vi "Create Enumeration.vi"(7 "App":refnum<vi>, 8 "error in (no error)":errorcluster, 10 "Enumeration":T1, 11 "LV-Protoc in":refnum<class "LV-Protoc.lvclass">) -> (0 "error out":errorcluster, 3 "LV-Protoc out":refnum<class "LV-Protoc.lvclass">)   [LabVIEW 2020, in "LV-Protoc.lvlib" / "LV-Protoc.lvclass"]
uses:
  LV-Protoc.lvclass
  LV-Proto/Enumeration.ctl
  LV-Proto/Enum Value.ctl
  LV-Protoc.lvlib
  LV-Proto/LV-Proto.lvlib
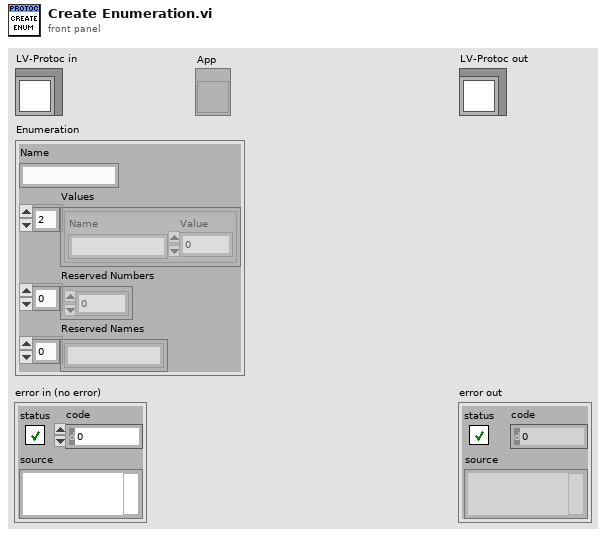
[diagram p1: front panel]
types:
  T1 = typedef "LV-Proto.lvlib/Enumeration.ctl" = cluster{"Name":string, "Values":T2[], "Reserved Numbers":u32[], "Reserved Names":string[]}
  T2 = typedef "LV-Proto.lvlib/Enum Value.ctl" = cluster{"Name":string, "Value":i32}
  T3 = typedef "LV-Protoc.lvlib/Enumeration Paths.ctl" = cluster{"Name":string, "Library":path, "Typedef":path, "Encode":path, "Encode packed":path, "Decode":path, "Decode packed":path, "Enum Value":path, "Enum from Value":path}
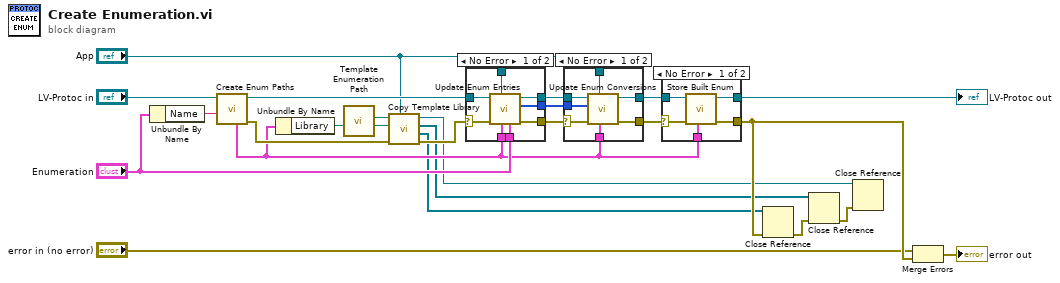
[diagram p0: block diagram]
diagram:
  n1 = Unbundle By Name("Enumeration") -> ("Name"=w14:string)
  n2 = call "Create Enum Paths.vi"("Enumeration Name"=w14, "LV-Protoc in"="LV-Protoc in") -> ("error out"=w13:errorcluster, "LV-Protoc out"=w15:refnum<class "LV-Protoc.lvclass">, "Enumeration Paths"=w8:T3)  [unwired: 7 in]
  n3 = Unbundle By Name(w8) -> ("Library"=w12:path)
  n4 = call "Template Enumeration Path.vi"() -> ("Template Enumeration Path"=w23:path)  [unwired: 11 in]
  n5 = call "Copy Template Library.vi"("App"="App", "error in (no error)"=w13, "Destination lvlib Path"=w12, "Source lvlib Path"=w23) -> ("error out"=w22:errorcluster, "Nested Libraries"=w5:refnum<vi>[], "VIs"=w3:refnum<vi>[], "Library"=w1:refnum<vi>)  [unwired: 4 in]
  n6 = case shown="No Error" w22 {
    selector: w22 -> [w30 w33]
    tunnel: w15 -> [w32 w34]
    tunnel: [w31 w34] -> w18
    tunnel: [w29 w33] -> w17
    tunnel: [w28 _] -> w16
    tunnel: "Enumeration" -> [w27 _]
    tunnel: w8 -> [w26 _]
    tunnel: "App" -> [w25 _]
    frame No Error {
      n7 = call "Update Enum Entries.vi"("Enumeration"=w27, "Built Enumeration"=w26, "App"=w25, "error in (no error)"=w30, "LV-Protoc in"=w32) -> ("error out"=w29:errorcluster, "Values"=w28:i32[], "LV-Protoc out"=w31:refnum<class "LV-Protoc.lvclass">)  [unwired: 4 in]
    }
    frame Error {
    }
  }
  n8 = case shown="No Error" w17 {
    selector: w17 -> [w39 w42]
    tunnel: w18 -> [w41 w43]
    tunnel: [w40 w43] -> w9
    tunnel: [w38 w42] -> w10
    tunnel: w16 -> [w37 _]
    tunnel: w8 -> [w36 _]
    tunnel: "App" -> [w35 _]
    frame No Error {
      n9 = call "Update Enum Conversions.vi"("Built Enumeration"=w36, "App"=w35, "error in (no error)"=w39, "Values"=w37, "LV-Protoc in"=w41) -> ("error out"=w38:errorcluster, "LV-Protoc out"=w40:refnum<class "LV-Protoc.lvclass">)  [unwired: 5 in]
    }
    frame Error {
    }
  }
  n10 = case shown="No Error" w10 {
    selector: w10 -> [w46 w49]
    tunnel: w9 -> [w48 w50]
    tunnel: [w47 w50] -> w7
    tunnel: [w45 w49] -> w24
    tunnel: w8 -> [w44 _]
    frame No Error {
      n11 = call "Store Built Enum.vi"("Built Enumeration"=w44, "error in (no error)"=w46, "LV-Protoc in"=w48) -> ("error out"=w45:errorcluster, "LV-Protoc out"=w47:refnum<class "LV-Protoc.lvclass">)  [unwired: 7 in]
    }
    frame Error {
    }
  }
  "LV-Protoc out" <- w7
  n12 = Close Reference(reference=w5, error in (no error)=w24) -> (error out=w4:errorcluster)
  n13 = Close Reference(reference=w3, error in (no error)=w4) -> (error out=w2:errorcluster)
  n14 = Close Reference(reference=w1, error in (no error)=w2) -> ()  [unwired: 1 out]
  n15 = Merge Errors("error in (no error)", w24) -> (→"error out":errorcluster)
